vi "Generic - AI1.vi"(0 "MW100":refnum<visa-resource-name>="MW100", 2 "Semiphore":T1, 5 "Channel_Enum":T2=1 items=["4-20_OUT", "Pres_HI1", "Pres_HI2", "Pres_LOW", "Pres_PIN", "HEATER_TOP", "HEATER_BOT", "T_Shell", "FLOWMETER", "WATT_SENSE", "WH_TICK", "Tc_1", "Tc_2", "Tc_3", "Tc_4", "Tc_5", "Tc_6", "Tc_down", "T_Shell_2", "T_Shell_3", "T_Shell_4", "RTD_IN", "RTD_OUT", "RTD_AMB", "INTF_TEMPFLO", "INTF_READY", "INTF_START", "INTF_STOP", "DRM_LOW", "DRM_HIGH", "PWR_MAIN", "VLV_DUMP", "VLV_OUT", "VLV_IN", "WATT_HOURS", "FLOW(SAMPLE)", "GALLONS", "FLOW(GPM)", "FLOW_CALC_GAIN", "FLOW_CALC_OFFSET", "FLOW_CALC_THRESHOLD", "VLV_DUMP_2", "VLV_OUT_2", "VLV_IN_2", "VLV_DUMP_3", "VLV_OUT_3", "VLV_IN_3", "VLV_DUMP_4", "VLV_OUT_4", "VLV_IN_4", "CHAN_34", "CHAN_35", "CHAN_36"], 11 "Error In":errorcluster) -> (4 "dup VISA session":refnum<visa-resource-name>, 6 "Value":dbl, 15 "Error Out":errorcluster)   [LabVIEW 2012]
uses:
  ChannelSettings.ctl
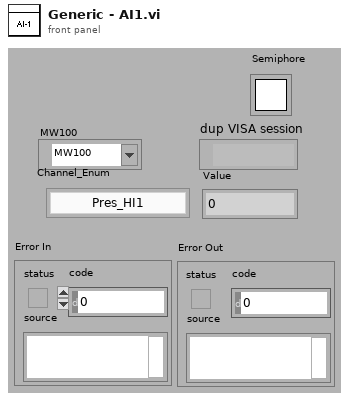
[diagram p1: front panel]
types:
  T1 = typedef "Semaphore RefNum" = refnum<k1>
  T2 = typedef "ChannelSettings.ctl" = u32
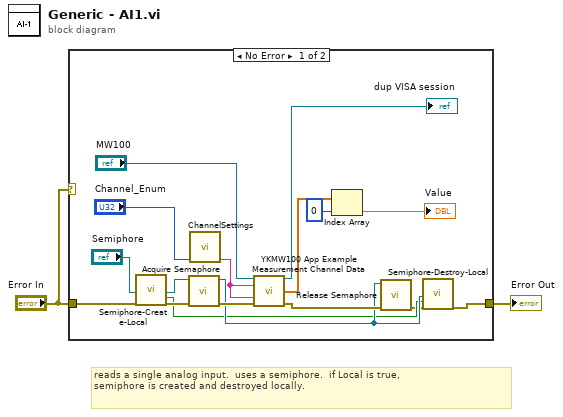
[diagram p0: block diagram]
diagram:
  # "reads a single analog input.  uses a semiphore.  if Local is true, \nsemiphore is created and destroyed locally."
  n1 = case shown="No Error" "Error In" {
    tunnel: "Error In" -> [w9 w20]
    tunnel: [w3 w20] -> w2
    frame No Error {
      n2 = call "Semiphore-Create-Local.vi"("Semiphore"="Semiphore", "error in (no error)"=w9) -> ("semaphore"=w8:T1, "Local?"=w5:bool, "error out"=w7:errorcluster)  [unwired: 15 in]
      n3 = call <vilib>:"Acquire Semaphore.vi"("error in (no error)"=w7, "semaphore"=w8) -> ("error out"=w13:errorcluster, "semaphore out"=w6:T1)  [unwired: 3 in, 1 out]
      n4 = call "ChannelSettings.vi"("Channel_Enum"="Channel_Enum") -> ("Channel String"=w19:string)  [unwired: 10 in]
      n5 = call "YKMW100 App Example Measurement Channel Data.vi"("VISA session"="MW100", "Start Channel (001)"=w19, "End Channel (001)"=w19, "error in (no error)"=w13) -> ("dup VISA session"=→"dup VISA session":refnum<visa-resource-name>, "Data List"=w16:dbl[], "error out"=w12:errorcluster)  [unwired: 4 in, 5 out]
      n6 = Index Array(array=w16, index=0) -> (element=→"Value":dbl)
      n7 = call <vilib>:"Release Semaphore.vi"("error in (no error)"=w12, "semaphore"=w6) -> ("error out"=w4:errorcluster)  [unwired: 4 in, 1 out]
      n8 = call "Semiphore-Destroy-Local.vi"("Semiphore"=w6, "Local?"=w5, "error in (no error)"=w4) -> ("error out"=w3:errorcluster)  [unwired: 16 in]
    }
    frame Error {
    }
  }
  "Error Out" <- w2
